vi "ConditionLux.vi"(3 "Offset":dbl min=0.0 max=5.0 step=0.01, 4 "Input":dbl) -> (0 "Underlimit":bool, 1 "Overlimit":bool)   [LabVIEW 2021]
panel:
  out "min offset":dbl
  out "max offset":dbl
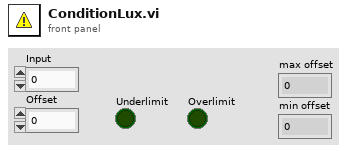
[diagram p1: front panel]
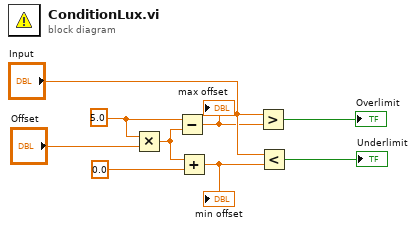
[diagram p0: block diagram]
diagram:
  w5 = 5.0 ("y")
  n1 = Multiply(x=w5, y="Offset") -> (x*y=w3:dbl)
  n2 = Subtract(x=w5, y=w3) -> (x-y=w1:dbl)
  "max offset" <- w1
  n3 = Add(x=w3, y=0.0) -> (x+y=w2:dbl)
  "min offset" <- w2
  n4 = Greater?(x="Input", y=w1) -> (0:→"Overlimit":bool)
  n5 = Less?(x="Input", y=w2) -> (x < y?=→"Underlimit":bool)
